vi "Measurement UI.vi"() -> ()   [LabVIEW 2023, in "FPT_SParam_VST UI.lvlib"]
uses:
  FPT_SParam_VST UI.lvlib
panel:
  in  "Tab Control 2":T1(tab)
  out "General Graph 1":T2(graph)
  out "General Graph 2":T2(graph)
  in  "Power sequencing file validity check":bool
  in  "Type of Stimulus":enum32{"CW", "Pulsed CW"}(ring)
  in  "Through Adapter S2P":string
  in  "Load S1P":string
  in  "Open S1P":string
  in  "Short S1P":string
  in  "Save Calibration File at":string
  in  "Calibration File Path":string
  in  "RFSG attenuation mode":enum32{"<None>", "Constant Attenuation"}(ring)=enum."Constant Attenuation"
  in  "RF In Switch":string
  in  "RF Out Switch":string
  in  "SnP File Path":string caption="SnP File Path (String)"
  in  "VST Resource Name":string="5842_0"
  in  "Power sequencing file path":string
  out "All Graph Refs":refnum<vi>[](array[refnum])
  out "S-Param Magnitude":dbl[][](array[numeric])
  out "S-Param Phase":dbl[][](array[numeric])
  out "S-Param":dbl[][](array[numeric])
  out "MeasTable":string[][](table)
  in  "Configuration":T3(ring)
  in  "Tab Control":T4(tab)
  in  "Power sequencing file path_update":path caption="Power Sequencing File Path"
  in  "Port2 Test":string
  in  "Port2 Reference":string
  in  "Port1 Test":string
  in  "Port1 Reference":string
  in  "RF In Switch_update":refnum<k15> caption="RF In Switch"
  in  "Port2 Incident":string
  in  "Port1 Incident":string
  in  "Common RFout":string
  in  "RF Out Switch_update":refnum<k15> caption="RF Out Switch"
  in  "Tab Control 3":enum32{"Calibrate", "Measure"}(tab)
  in  "Save Calibration Result_path":path caption="Save Calibration Result"
  in  "Short S1P_path":path caption="Short S1P"
  in  "Open S1P_path":path caption="Open S1P"
  in  "Load S1P_path":path caption="Load S1P"
  in  "Through Adapter S2P_path":path caption="Through Adapter S2P"
  in  "Calibration File Path_path":path caption="Calibration File Path"
  in  "RFSG attenuation mode_tab":enum32{"<None>", "Constant Attenuation"}(tab)=enum."Constant Attenuation" caption="RFSG Attenuation Mode"
  in  "RFSG external attenuation (dB)":dbl caption="External Attenuation" format="%#.3pdB"
  in  "VST name_update":refnum<k15> caption="VST Name"
  in  "RFSG port":string(combo)="port1" caption="RFSG Port"
  in  "RFmx port":string(combo)="port2" caption="RFmx Port"
  in  "SnP File Path_path":path caption="SnP File Path"
  in  "Step Size (Hz)":dbl=200.0 caption="Step Size" format="%#pHz"
  in  "Start Frequency (Hz)":dbl=4000000000.0 caption="Start Frequency" format="%#pHz"
  in  "Stop Frequency (Hz)":dbl=26000000000.0 caption="Stop Frequency" format="%#pHz"
  in  "IF Bandwidth (Hz)":dbl=100000.0 caption="IF Bandwidth" format="%#pHz"
  in  "External Gain (dB)":dbl caption="External Gain" format="%#fdB"
  in  "Power Level (dBm)":dbl=-10.0 caption="Power Level" format="%#fdBm"
  in  "Stimulus_tab":enum32{"CW", "Pulsed CW"}(tab)=enum."Pulsed CW" caption="Stimulus"
  in  "PRI (s)":dbl caption="PRI" format="%#.3ps"
  in  "Pulse Width (s)":dbl caption="Pulse Width" format="%#.3ps"
  in  "Average Mode":enum32{"Per Sweep", "Per Point"}(ring)
  in  "Number of Averages":i32=200
  in  "Action":enum32{"Calibrate", "Measure"}(ring)=enum."Measure"
  out "Status":string
  # "RFOut Switches"
  # "RFIn Switches"
  # "Calibration"
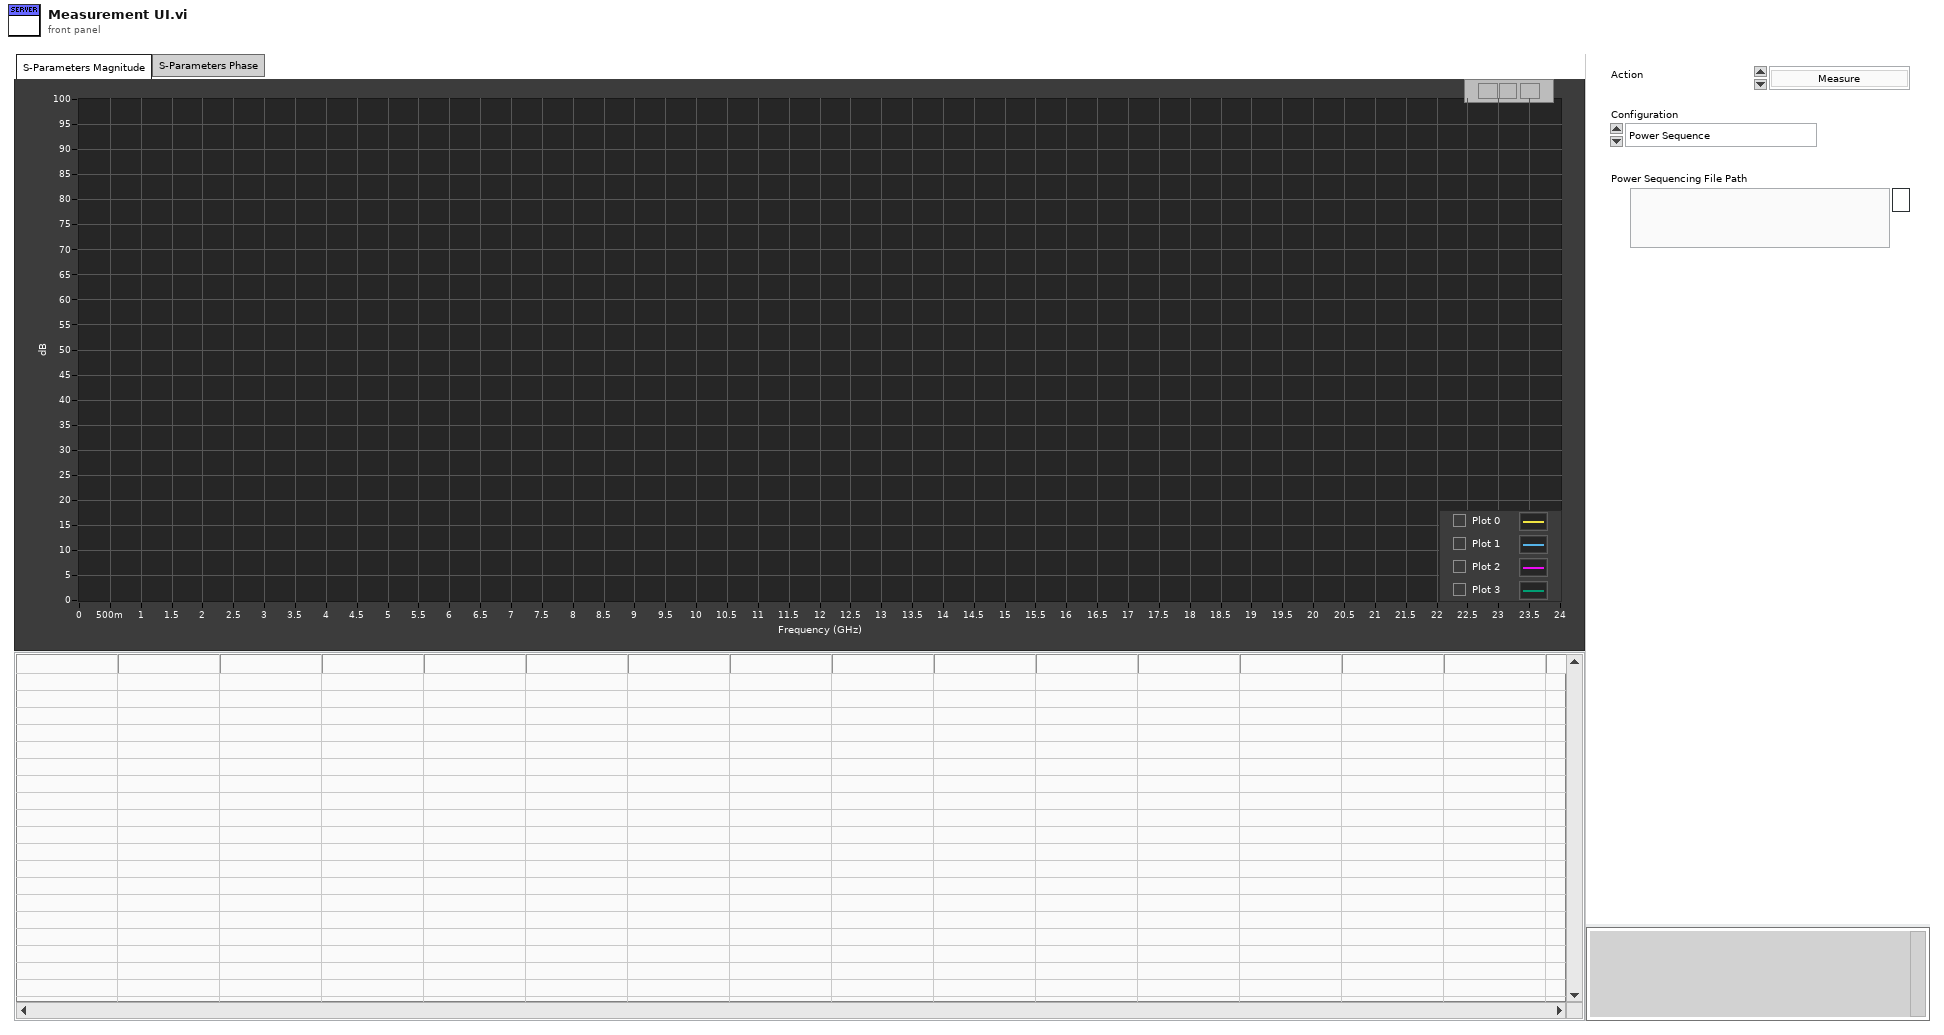
[diagram p1: front panel]
types:
  T1 = enum32{"S-Parameters Magnitude", "S-Parameters Phase", "Hiden Controls"}
  T2 = cluster{"Load currents":dbl[], "Efficiency":dbl[]}[]
  T3 = enum32{"Power Sequence", "Switches", "HW + Correction", "Measurement 1"}
  T4 = enum32{"Power Sequence", "Switches", "Correction", "Measurement 1"}
  T5 = cluster{"Shift":bool, "Ctrl":bool, "Alt":bool, "Cmd":bool, "Opt":bool}
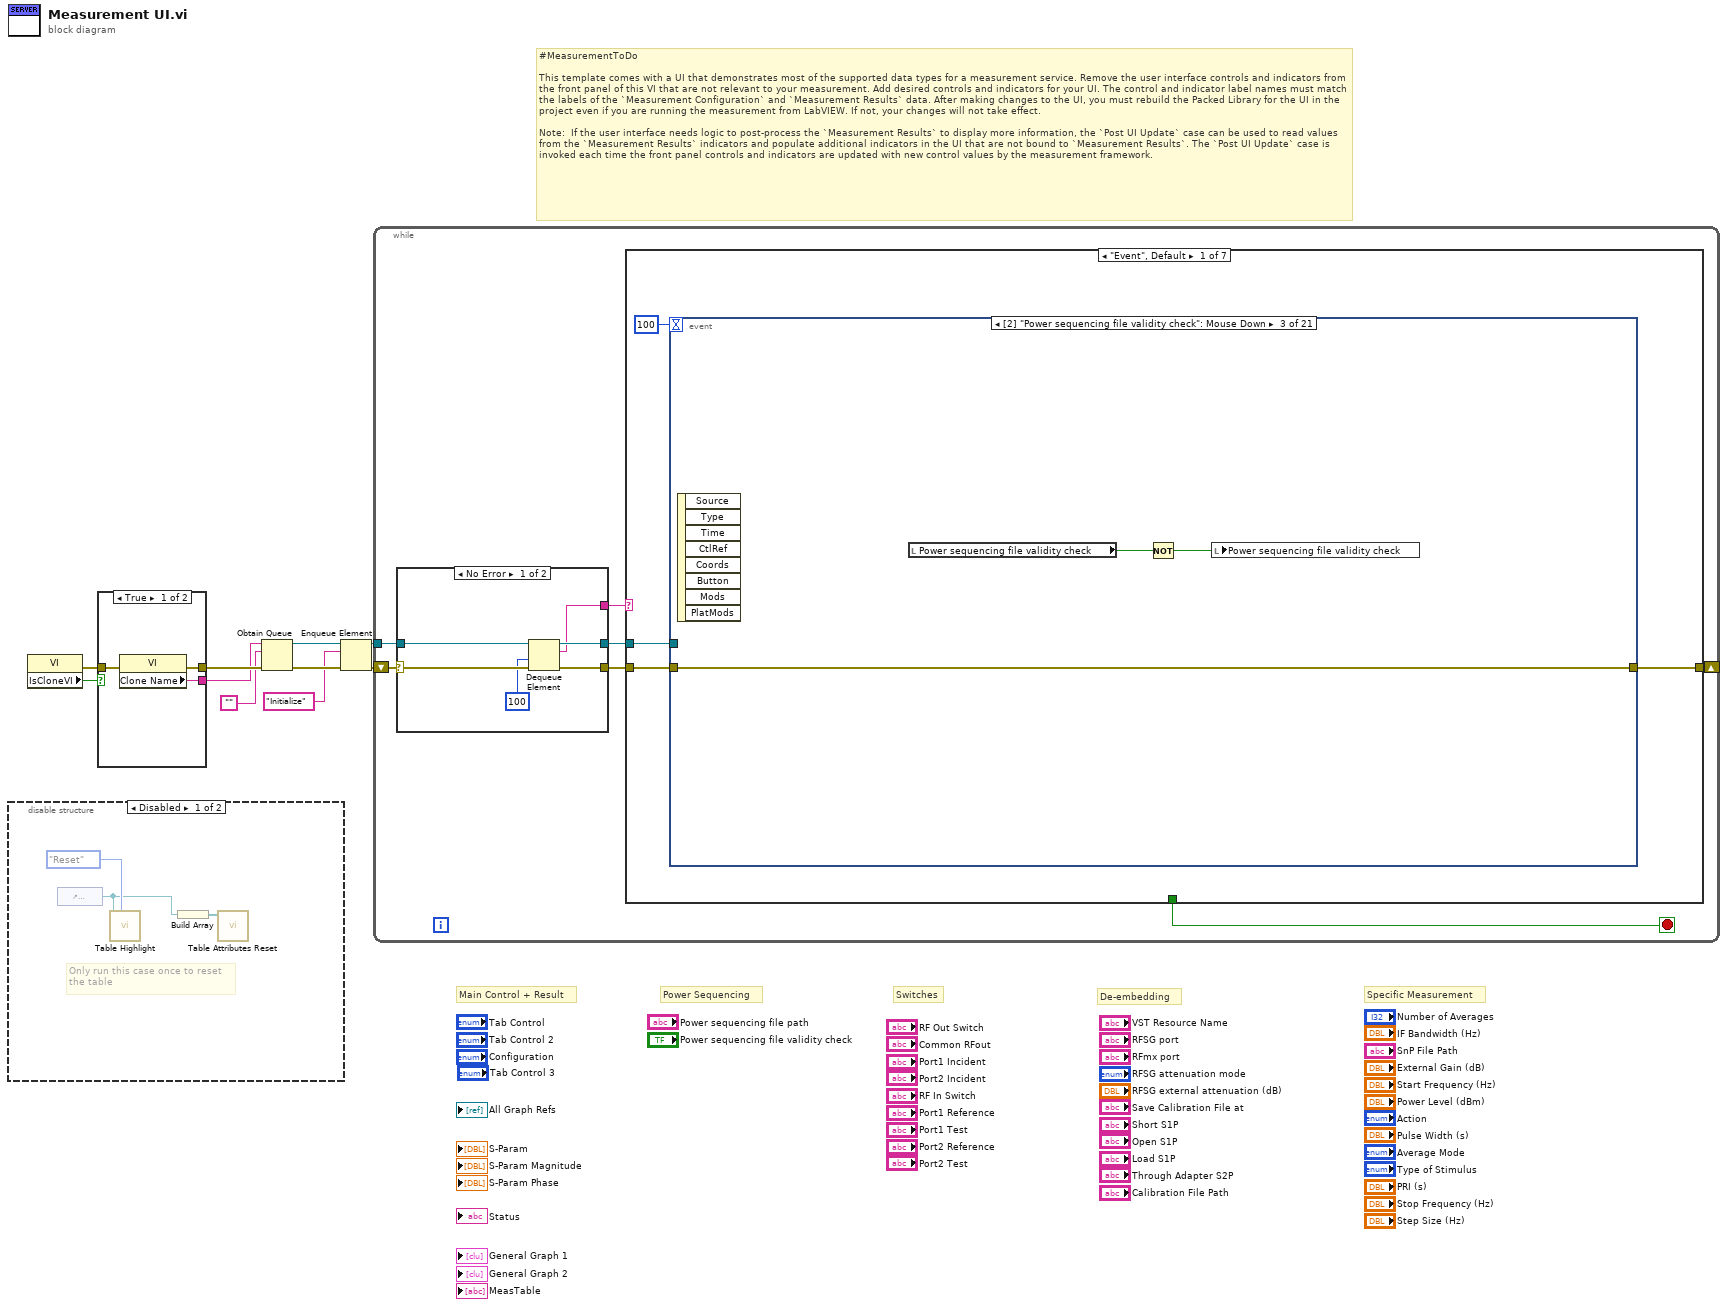
[diagram p0: block diagram]
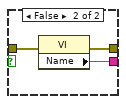
[diagram p3: hidden frame]
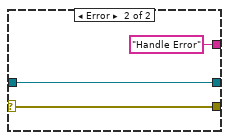
[diagram p4: hidden frame]
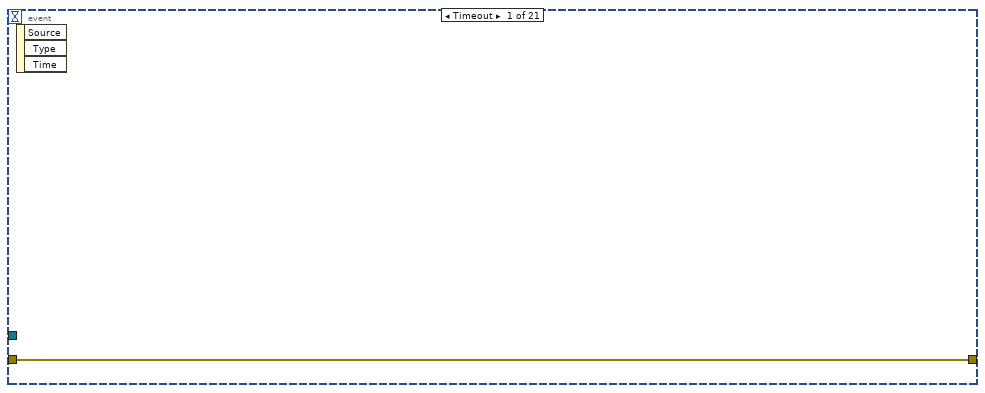
[diagram p5: hidden frame]
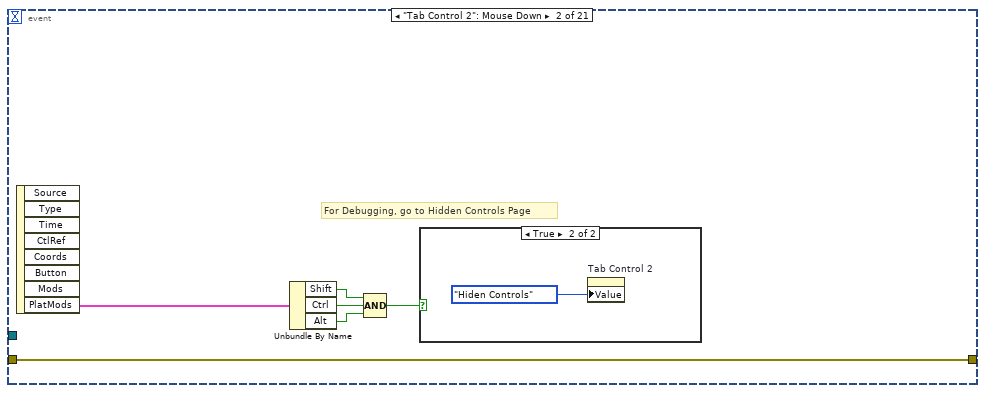
[diagram p6: hidden frame]
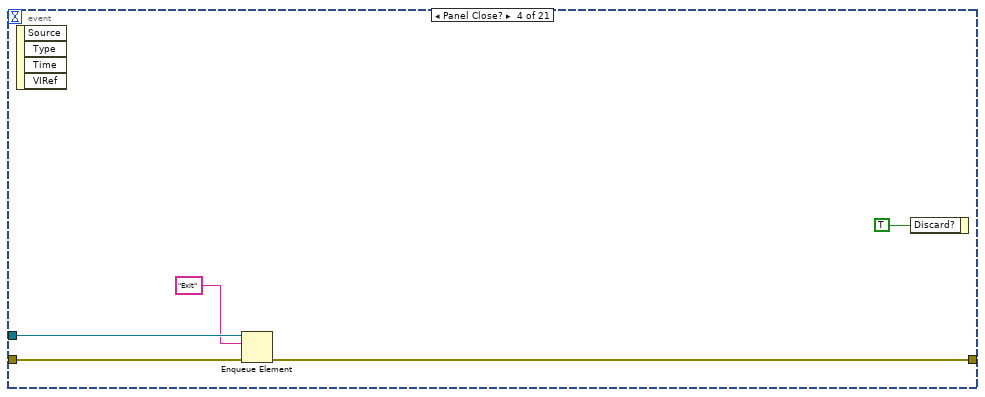
[diagram p8: hidden frame]
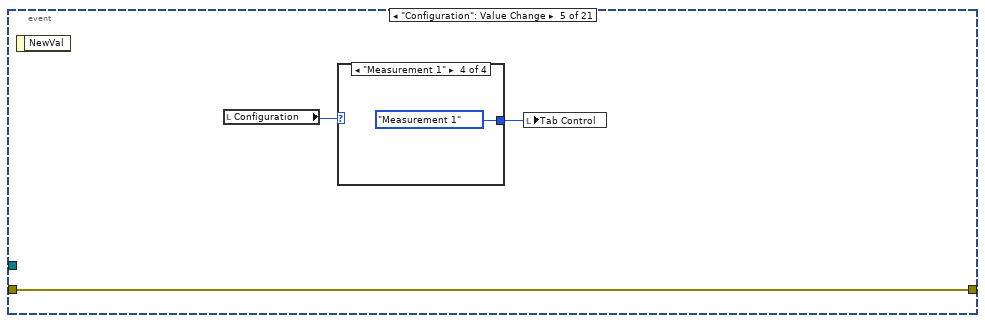
[diagram p9: hidden frame]
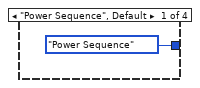
[diagram p10: hidden frame]
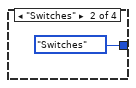
[diagram p11: hidden frame]
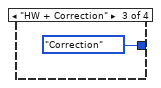
[diagram p12: hidden frame]
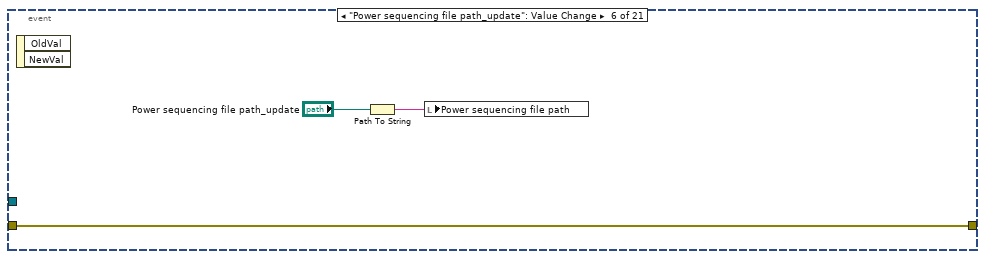
[diagram p13: hidden frame]
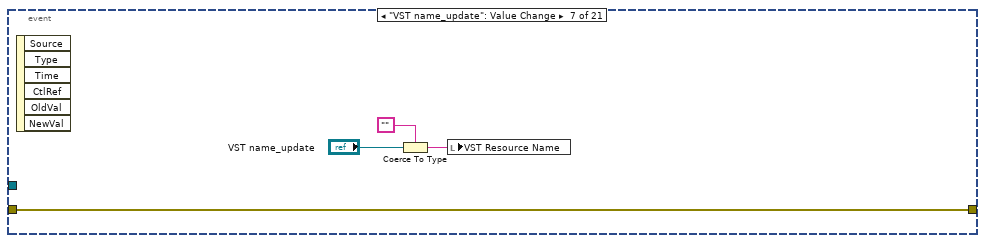
[diagram p14: hidden frame]
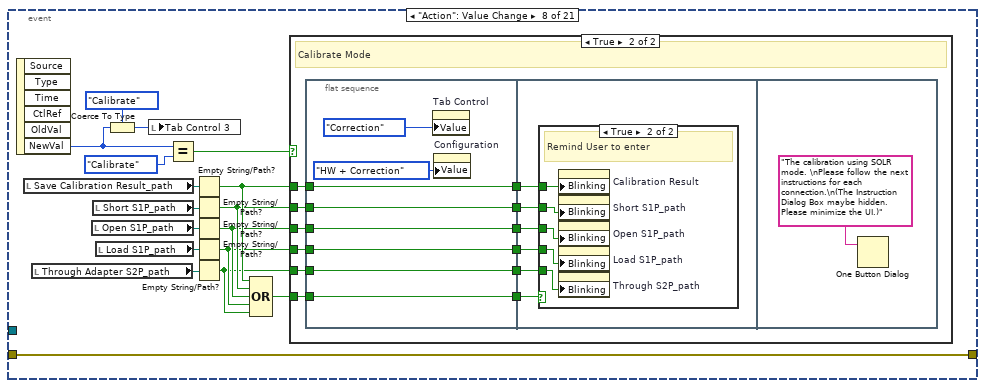
[diagram p15: hidden frame]
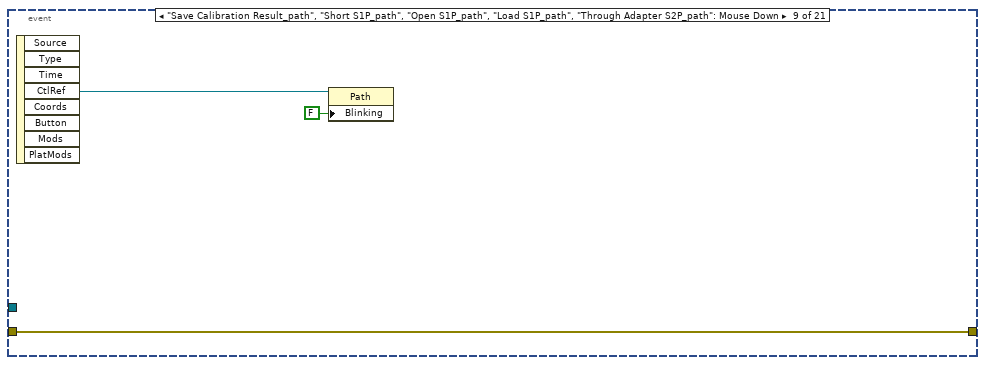
[diagram p18: hidden frame]
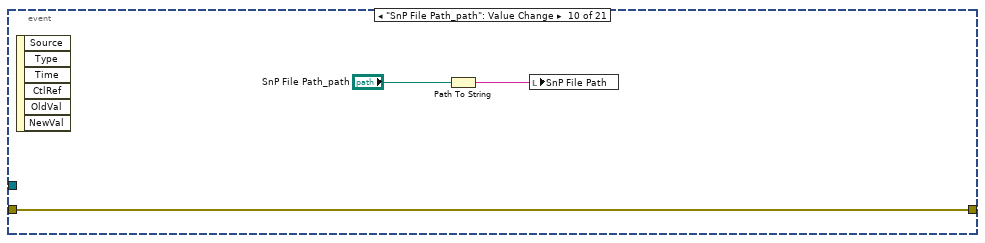
[diagram p19: hidden frame]
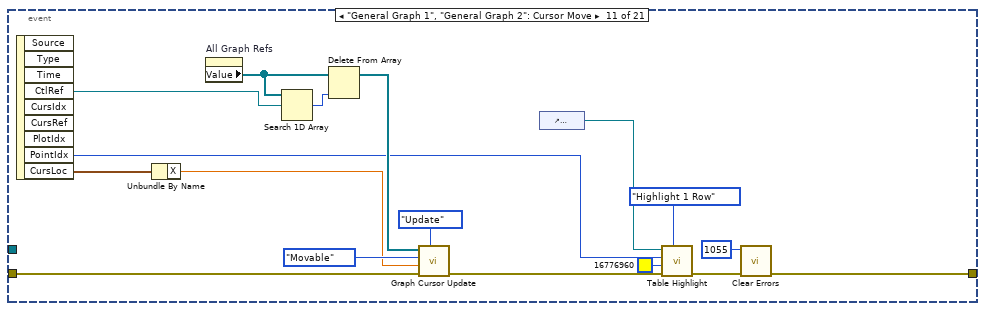
[diagram p20: hidden frame]
diagram:
  # "Switches"
  # "Specific Measurement"
  # "De-embedding"
  # "Power Sequencing"
  # "Main Control + Result"
  # "#MeasurementToDo  \n\nThis template comes with a UI that demonstrates most of the supported data types for a measurement service. Remove the user interface controls and indicators from the front panel of this VI that are not relevant to your measurement. Add desired controls and indicators for your UI. The control and indicator label names must match the labels of the `Measurement Configuration` and `Measurement Results` data. After making changes to the UI, you must rebuild the Packed Library for the UI in the project even if you are running the measurement from LabVIEW. If not, your changes will not take effect.\n\nNote:  If the user interface needs logic to post-process the `Measurement Results` to display more information, the `Post UI Update` case can be used to read values from the `Measurement Results` indicators and populate additional indicators in the UI that are not bound to `Measurement Results`. The `Post UI Update` case is invoked each time the front panel controls and indicators are updated with new control values by the measurement framework."
  n1 = disable-structure shown="Disabled" {
    frame Disabled {
      # "Only run this case once to reset\nthe table"
      n2 = control-ref of="MeasTable"() -> (w11:refnum<vi>)
      n3 = call "Table Highlight.vi"("Action"=enum16{"Reset", "Highlight 1 Row"}."Reset", "Table Ref in"=w11) -> ()  [unwired: 8 in, 2 out]
      n4 = Build Array(w11) -> (w12:refnum<vi>[])
      n5 = call "Table Attributes Reset.vi"("Table Refs"=w12) -> ()  [unwired: 11 in]
    }
    frame Enabled {
    }
  }
  n6 = property class="VI"() -> (error out=w1:errorcluster, "IsCloneVI"=w2:bool)  [unwired: 2 in, 1 out]
  n7 = case shown="True" w2 {
    tunnel: [w16 w19] -> w10
    tunnel: [w15 w18] -> w9
    tunnel: w1 -> [w14 w17]
    frame True {
      n8 = property class="VI"(error in=w14) -> (error out=w16:errorcluster, "Clone Name"=w15:string)  [unwired: 1 in, 1 out]
    }
    frame False {
      n9 = property class="VI"(error in=w17) -> (error out=w19:errorcluster, "Name"=w18:string)  [unwired: 1 in, 1 out]
    }
  }
  n10 = Obtain Queue(name (unnamed)=w9, element data type="", error in (no error)=w10) -> (queue out=w6:refnum<queue>, error out=w8:errorcluster)  [unwired: 2 in, 1 out]
  n11 = Enqueue Element(queue=w6, element="Initialize", error in (no error)=w8) -> (queue out=w5:refnum<queue>, error out=w7:errorcluster)  [unwired: 1 in, 1 out]
  n12 = while {
    shift-right: [w21] -> _
    shift-left: w7 -> [w26]
    tunnel: w5 -> [w24]
    stop <- w20 stop-if-true
    n13 = case shown="No Error" w26 {
      selector: w26 -> [w32 w35]
      tunnel: [w31 w35] -> w25
      tunnel: w24 -> [w30 w34]
      tunnel: [w29 w34] -> w23
      tunnel: [w28 "Handle Error"] -> w22
      frame No Error {
        n14 = Dequeue Element(queue=w30, timeout in ms (-1)=100, error in (no error)=w32) -> (queue out=w29:refnum<queue>, element=w28:string, error out=w31:errorcluster)  [unwired: 1 out]
      }
      frame Error {
      }
    }
    n15 = case shown="\"Event\", Default" w22 {
      tunnel: w25 -> [w38 w182 w219 w236 w247 w254 w255]
      tunnel: w23 -> [w36 _ w218 w235 _ w252 _]
      tunnel: [w39 w182 w219 w237 w246 w249 w255] -> w21
      tunnel: [_ _ _ _ _ TRUE _] -> w20
      frame "Event", Default {
        n16 = event shown="[2] \"Power sequencing file validity check\": Mouse Down" {
          selector: _ -> [_ _ _ _ _ _ _ _ _ _ _ _ _ _ _ _ _ _ _ _ _]
          dyn-events: _ -> [_ _ _ _ _ _ _ _ _ _ _ _ _ _ _ _ _ _ _ _ _]
          timeout: 100 -> [_ _ _ _ _ _ _ _ _ _ _ _ _ _ _ _ _ _ _ _ _]
          tunnel: [w40 w46 w50 w53 w58 w63 w66 w86 w121 w124 w134 w145 w149 w153 w156 w159 w162 w165 w168 w171 w175] -> w39
          tunnel: w38 -> [w40 w46 w50 w54 w58 w63 w66 w86 w121 w124 w135 w145 w149 w153 w156 w159 w162 w165 w168 w171 w175]
          tunnel: w36 -> [_ _ _ w52 _ _ _ _ _ _ _ _ _ _ _ _ _ _ _ _ _]
          event Timeout {
            n17 = event-data() -> ()  [unwired: 1 in, 3 out]
          }
          event "Tab Control 2": Mouse Down {
            # "For Debugging, go to Hidden Controls Page"
            n18 = event-data() -> ("PlatMods"=w45:T5)  [unwired: 1 in, 7 out]
            n19 = Unbundle By Name(w45) -> ("Shift"=w44:bool, "Ctrl"=w43:bool, "Alt"=w42:bool)
            n20 = Compound Arithmetic op=AND(w44, w43, w42) -> (w41:bool)
            n21 = case shown="True" w41 {
              frame False {
              }
              frame True {
                n22 = property on="Tab Control 2" class="TabCtl (strict)"("Value"=T1."Hiden Controls" ("Tab Control 2")) -> ()  [unwired: 2 in, 2 out]
              }
            }
          }
          event "Power sequencing file validity check": Mouse Down {
            n23 = event-data() -> ()  [unwired: 1 in, 8 out]
            n24 = local read "Power sequencing file validity check"() -> (w49:bool)
            n25 = Not(x=w49) -> (.not. x?=w48:bool)
            n26 = local write "Power sequencing file validity check"(w48) -> ()
          }
          event Panel Close? {
            n27 = event-data() -> ()  [unwired: 1 in, 4 out]
            n28 = Enqueue Element(queue=w52, element="Exit", error in (no error)=w54) -> (error out=w53:errorcluster)  [unwired: 1 in, 2 out]
            n29 = event-data("Discard?"=TRUE) -> ()  [unwired: 1 in, 1 out]
          }
          event "Configuration": Value Change {
            n30 = event-data() -> ()  [unwired: 1 in, 1 out]
            n31 = local read "Configuration"() -> (w56:T3)
            n32 = case shown="\"Measurement 1\"" w56 {
              tunnel: [T4."Power Sequence" ("Tab Control") T4."Switches" ("Tab Control") T4."Correction" ("Tab Control") T4."Measurement 1" ("Tab Control")] -> w57
              frame "Power Sequence", Default {
              }
              frame "Switches" {
              }
              frame "HW + Correction" {
              }
              frame "Measurement 1" {
              }
            }
            n33 = local write "Tab Control"(w57) -> ()
          }
          event "Power sequencing file path_update": Value Change {
            n34 = event-data() -> ()  [unwired: 1 in, 2 out]
            n35 = Path To String(path="Power sequencing file path_update") -> (string=w64:string)
            n36 = local write "Power sequencing file path"(w64) -> ()
          }
          event "VST name_update": Value Change {
            n37 = event-data() -> ()  [unwired: 1 in, 6 out]
            n38 = Coerce To Type(0:"VST name_update", 1:"") -> (2:w68:string)
            n39 = local write "VST Resource Name"(w68) -> ()
          }
          event "Action": Value Change {
            n40 = event-data() -> ("NewVal"=w83:enum32{"Calibrate", "Measure"})  [unwired: 1 in, 5 out]
            n41 = local read "Save Calibration Result_path"() -> (w80:path)
            n42 = local read "Through Adapter S2P_path"() -> (w76:path)
            n43 = local read "Open S1P_path"() -> (w78:path)
            n44 = local read "Short S1P_path"() -> (w79:path)
            n45 = local read "Load S1P_path"() -> (w77:path)
            n46 = Coerce To Type(0:w83, 1:enum32{"Calibrate", "Measure"}."Calibrate" ("Tab Control 3")) -> (2:w81:enum32{"Calibrate", "Measure"})
            n47 = local write "Tab Control 3"(w81) -> ()
            n48 = Equal?(x=w83, y=enum32{"Calibrate", "Measure"}."Calibrate") -> (x = y?=w84:bool)
            n49 = Empty String/Path?(string/path=w80) -> (empty?=w75:bool)
            n50 = Empty String/Path?(string/path=w79) -> (empty?=w74:bool)
            n51 = Empty String/Path?(string/path=w78) -> (empty?=w73:bool)
            n52 = Empty String/Path?(string/path=w77) -> (empty?=w72:bool)
            n53 = Empty String/Path?(string/path=w76) -> (empty?=w71:bool)
            n54 = Compound Arithmetic op=OR(w75, w74, w73, w72, w71) -> (w70:bool)
            n55 = case shown="True" w84 {
              tunnel: w75 -> [_ w97]
              tunnel: w74 -> [_ w95]
              tunnel: w73 -> [_ w93]
              tunnel: w72 -> [_ w91]
              tunnel: w71 -> [_ w89]
              tunnel: w70 -> [_ w87]
              frame False {
                # "Measure Mode"
              }
              frame True {
                # "Calibrate Mode"
                n56 = flat-sequence {
                  tunnel: [w105] -> w98
                  tunnel: w97 -> [w105]
                  tunnel: [w104] -> w96
                  tunnel: w95 -> [w104]
                  tunnel: [w103] -> w94
                  tunnel: w93 -> [w103]
                  tunnel: [w102] -> w92
                  tunnel: w91 -> [w102]
                  tunnel: [w101] -> w90
                  tunnel: w89 -> [w101]
                  tunnel: [w100] -> w88
                  tunnel: w87 -> [w100]
                  tunnel: w98 -> [w112]
                  tunnel: w96 -> [w111]
                  tunnel: w94 -> [w110]
                  tunnel: w92 -> [w109]
                  tunnel: w90 -> [w108]
                  tunnel: w88 -> [w107]
                  frame #0 {
                    n57 = property on="Tab Control" class="TabCtl (strict)"("Value"=T4."Correction" ("Tab Control")) -> ()  [unwired: 2 in, 2 out]
                    n58 = property on="Configuration" class="Enum (strict)"("Value"=T3."HW + Correction" ("Configuration")) -> ()  [unwired: 2 in, 2 out]
                  }
                  frame #1 {
                    n59 = case shown="True" w107 {
                      tunnel: w112 -> [_ w117]
                      tunnel: w111 -> [_ w116]
                      tunnel: w110 -> [_ w115]
                      tunnel: w109 -> [_ w114]
                      tunnel: w108 -> [_ w113]
                      frame False {
                      }
                      frame True {
                        # "Remind User to enter"
                        n60 = property on="Calibration Result" class="Path"("Blinking"=w117) -> ()  [unwired: 2 in, 2 out]
                        n61 = property on="Short S1P_path" class="Path"("Blinking"=w116) -> ()  [unwired: 2 in, 2 out]
                        n62 = property on="Open S1P_path" class="Path"("Blinking"=w115) -> ()  [unwired: 2 in, 2 out]
                        n63 = property on="Load S1P_path" class="Path"("Blinking"=w114) -> ()  [unwired: 2 in, 2 out]
                        n64 = property on="Through S2P_path" class="Path"("Blinking"=w113) -> ()  [unwired: 2 in, 2 out]
                      }
                    }
                  }
                  frame #2 {
                    n65 = One Button Dialog(message="The calibration using SOLR mode. \nPlease follow the next instructions for each connection.\n(The Instruction Dialog Box maybe hidden. Please minimize the UI.)") -> ()  [unwired: 1 in, 1 out]
                  }
                }
              }
            }
          }
          event "Save Calibration Result_path", "Short S1P_path", "Open S1P_path", "Load S1P_path", "Through Adapter S2P_path": Mouse Down {
            n66 = event-data() -> ("CtlRef"=w120:refnum<vi>)  [unwired: 1 in, 7 out]
            n67 = property class="Path"(reference=w120, "Blinking"=FALSE) -> ()  [unwired: 1 in, 2 out]
          }
          event "SnP File Path_path": Value Change {
            n68 = event-data() -> ()  [unwired: 1 in, 6 out]
            n69 = Path To String(path="SnP File Path_path") -> (string=w122:string)
            n70 = local write "SnP File Path"(w122) -> ()
          }
          event "General Graph 1", "General Graph 2": Cursor Move {
            n71 = event-data() -> ("CtlRef"=w125:refnum<vi>, "PointIdx"=w128:i32, "CursLoc"=w133:cluster{"X":dbl, "Y":dbl})  [unwired: 1 in, 6 out]
            n72 = Unbundle By Name(w133) -> ("X"=w132:dbl)
            n73 = property on="All Graph Refs" class="Arr (strict)"() -> ("Value"=w129:refnum<vi>[])  [unwired: 2 in, 2 out]
            n74 = Search 1D Array(1D array=w129, element=w125) -> (index of element=w131:i32)  [unwired: 1 in]
            n75 = Delete From Array(array=w129, index=w131) -> (array with subset deleted=w130:refnum<vi>[])  [unwired: 1 in, 1 out]
            n76 = call "Graph Cursor Update.vi"("Action"=enum16{"Reset", "Update"}."Update" ("Cursor to Update"), "error in"=w135, "New X position"=w132, "Cursor Type"=enum16{"Movable", "Fixed", "All"}."Movable", "Graph Refs in"=w130) -> ("error out"=w138:errorcluster)  [unwired: 5 in, 1 out]
            n77 = control-ref of="MeasTable"() -> (w127:refnum<vi>)
            n78 = call "Table Highlight.vi"("Action"=enum16{"Reset", "Highlight 1 Row"}."Highlight 1 Row", "error in"=w138, "Color Box"=u32 16776960, "Row"=w128, "Table Ref in"=w127) -> ("error out"=w140:errorcluster)  [unwired: 5 in, 1 out]
            n79 = call <vilib>:"Clear Errors.vi"("error in (no error)"=w140, "specific error code to clear (0: all)"=1055) -> ("error out"=w134:errorcluster)  [unwired: 4 in, 1 out]
          }
          event "RF Out Switch_update": Value Change {
            n80 = event-data() -> ()  [unwired: 1 in, 6 out]
            n81 = Coerce To Type(0:"RF Out Switch_update", 1:"") -> (2:w143:string)
            n82 = local write "RF Out Switch"(w143) -> ()
          }
          event "RF In Switch_update": Value Change {
            n83 = event-data() -> ()  [unwired: 1 in, 6 out]
            n84 = Coerce To Type(0:"RF In Switch_update", 1:"") -> (2:w147:string)
            n85 = local write "RF In Switch"(w147) -> ()
          }
          event "RFSG attenuation mode_tab": Value Change {
            n86 = event-data() -> ()  [unwired: 1 in, 6 out]
            n87 = Coerce To Type(0:"RFSG attenuation mode_tab", 1:enum32{"<None>", "Constant Attenuation"}."<None>" ("RFSG attenuation mode")) -> (2:w151:enum32{"<None>", "Constant Attenuation"})
            n88 = local write "RFSG attenuation mode"(w151) -> ()
          }
          event "Save Calibration Result_path": Value Change {
            n89 = event-data() -> ()  [unwired: 1 in, 6 out]
            n90 = Path To String(path="Save Calibration Result_path") -> (string=w154:string)
            n91 = local write "Save Calibration File at"(w154) -> ()
          }
          event "Short S1P_path": Value Change {
            n92 = event-data() -> ()  [unwired: 1 in, 6 out]
            n93 = Path To String(path="Short S1P_path") -> (string=w158:string)
            n94 = local write "Short S1P"(w158) -> ()
          }
          event "Open S1P_path": Value Change {
            n95 = event-data() -> ()  [unwired: 1 in, 6 out]
            n96 = Path To String(path="Open S1P_path") -> (string=w161:string)
            n97 = local write "Open S1P"(w161) -> ()
          }
          event "Load S1P_path": Value Change {
            n98 = event-data() -> ()  [unwired: 1 in, 6 out]
            n99 = Path To String(path="Load S1P_path") -> (string=w164:string)
            n100 = local write "Load S1P"(w164) -> ()
          }
          event "Through Adapter S2P_path": Value Change {
            n101 = event-data() -> ()  [unwired: 1 in, 6 out]
            n102 = Path To String(path="Through Adapter S2P_path") -> (string=w167:string)
            n103 = local write "Through Adapter S2P"(w167) -> ()
          }
          event "Calibration File Path_path": Value Change {
            n104 = event-data() -> ()  [unwired: 1 in, 6 out]
            n105 = Path To String(path="Calibration File Path_path") -> (string=w170:string)
            n106 = local write "Calibration File Path"(w170) -> ()
          }
          event "Stimulus_tab": Value Change {
            n107 = event-data() -> ()  [unwired: 1 in, 6 out]
            n108 = Coerce To Type(0:"Stimulus_tab", 1:enum16{"CW", "Pulsed CW"}."CW" ("Type of Stimulus")) -> (2:w172:enum16{"CW", "Pulsed CW"})
            n109 = local write "Type of Stimulus"(w172) -> ()
          }
        }
      }
      frame "Initialize" {
        w176 = enum32{"Calibrate", "Measure"}."Measure" ("Action")
        w177 = 0
        n110 = control-ref of="General Graph 1"() -> (w180:refnum<vi>)
        n111 = control-ref of="General Graph 2"() -> (w178:refnum<vi>)
        n112 = local write "Tab Control"(w177) -> ()
        n113 = local write "Configuration"(w177) -> ()
        n114 = local write "Tab Control 2"(w177) -> ()
        n115 = local write "Action"(w176) -> ()
        n116 = local write "Tab Control 3"(w176) -> ()
        n117 = Build Array(w180, w178) -> (w179:refnum<vi>[])
        n118 = property on="All Graph Refs" class="Arr (strict)"("Value"=w179) -> ()  [unwired: 2 in, 2 out]
        n119 = call "Graph Set Cursor Mode.vi"("Cursor Mode"=enum32{"Free-Drag", "Single-Plot", "Multi-Plot"}."Multi-Plot", "Graph Refs in"=w179) -> ()  [unwired: 8 in, 2 out]
      }
      frame "Post UI Update" {
        # "This case will be triggered, after framework updates the User interface with result values.\nUsed to update data type def"
        n120 = local read "Power sequencing file path"() -> (w215:string)
        n121 = local read "Save Calibration File at"() -> (w209:string)
        n122 = local read "Through Adapter S2P"() -> (w189:string)
        n123 = local read "Calibration File Path"() -> (w186:string)
        n124 = local read "SnP File Path"() -> (w208:string)
        n125 = Enqueue Element(queue=w218, element="Post UI Update 2") -> ()  [unwired: 2 in, 3 out]
        n126 = local read "Open S1P"() -> (w205:string)
        n127 = local read "Short S1P"() -> (w214:string)
        n128 = local read "Load S1P"() -> (w190:string)
        n129 = String To Path(string=w190) -> (path=w191:path)
        n130 = String To Path(string=w189) -> (path=w188:path)
        n131 = String To Path(string=w186) -> (path=w187:path)
        n132 = String To Path(string=w215) -> (path=w216:path)
        n133 = String To Path(string=w209) -> (path=w206:path)
        n134 = String To Path(string=w208) -> (path=w207:path)
        n135 = String To Path(string=w205) -> (path=w204:path)
        n136 = String To Path(string=w214) -> (path=w213:path)
        n137 = local write "Power sequencing file path_update"(w216) -> ()
        n138 = local write "Save Calibration Result_path"(w206) -> ()
        n139 = local write "SnP File Path_path"(w207) -> ()
        n140 = local write "Open S1P_path"(w204) -> ()
        n141 = local write "Short S1P_path"(w213) -> ()
        n142 = local write "Load S1P_path"(w191) -> ()
        n143 = local write "Through Adapter S2P_path"(w188) -> ()
        n144 = local write "Calibration File Path_path"(w187) -> ()
        n145 = local read "RFSG attenuation mode"() -> (w197:enum32{"<None>", "Constant Attenuation"})
        n146 = local read "VST Resource Name"() -> (w210:string)
        n147 = local read "Type of Stimulus"() -> (w193:enum32{"CW", "Pulsed CW"})
        n148 = local read "RF Out Switch"() -> (w203:string)
        n149 = local read "RF In Switch"() -> (w198:string)
        n150 = local read "Action"() -> (w184:enum32{"Calibrate", "Measure"})
        n151 = Coerce To Type(0:w203, 1:refnum<k15> refnum ("RFSG name_update")) -> (2:w201:refnum<k15>)
        n152 = Coerce To Type(0:w198, 1:refnum<k15> refnum ("RFSG name_update")) -> (2:w200:refnum<k15>)
        n153 = Coerce To Type(0:w184, 1:enum32{"Calibrate", "Measure"}."Calibrate" ("Tab Control 3")) -> (2:w183:enum32{"Calibrate", "Measure"})
        n154 = Coerce To Type(0:w210, 1:refnum<k15> refnum ("RFSG name_update")) -> (2:w212:refnum<k15>)
        n155 = Coerce To Type(0:w197, 1:enum32{"<None>", "Constant Attenuation"}."Constant Attenuation" ("RFSG attenuation mode_tab")) -> (2:w196:enum32{"<None>", "Constant Attenuation"})
        n156 = Coerce To Type(0:w193, 1:enum32{"CW", "Pulsed CW"}."CW" ("Stimulus_tab")) -> (2:w194:enum32{"CW", "Pulsed CW"})
        n157 = local write "RF Out Switch_update"(w201) -> ()
        n158 = local write "RFSG attenuation mode_tab"(w196) -> ()
        n159 = local write "VST name_update"(w212) -> ()
        n160 = local write "RF In Switch_update"(w200) -> ()
        n161 = local write "Stimulus_tab"(w194) -> ()
        n162 = local write "Tab Control 3"(w183) -> ()
      }
      frame "Post UI Update 2" {
        w221 = string[] ["S11(deg)", "S21(deg)", "S12(deg)", "S22(deg)"] ("Plot Names")
        w222 = string[] ["S11(dB)", "S21(dB)", "S12(dB)", "S22(dB)"] ("Plot Names")
        # "Phase Graph"
        # "Mag Graph"
        # "Run after Post UI Update. Can be duplicate is need more processing.\nUtilize this case to convert the result to graph or table"
        n163 = Enqueue Element(queue=w235, element="Post UI Update 3", error in (no error)=w236) -> (error out=w237:errorcluster)  [unwired: 1 in, 2 out]
        n164 = control-ref of="General Graph 1"() -> (w234:refnum<vi>)
        n165 = property on="S-Param Magnitude" class="Arr (strict)"() -> ("Value"=w231:dbl[][])  [unwired: 2 in, 2 out]
        n166 = control-ref of="General Graph 2"() -> (w232:refnum<vi>)
        n167 = property on="S-Param Phase" class="Arr (strict)"() -> ("Value"=w228:dbl[][])  [unwired: 2 in, 2 out]
        n168 = call "Graph Assign Plot Names and Data.vi"("Legend Number of Rows"=4, "X Ys Data"=w231, "Plot Names"=w222, "Graph Ref in"=w234) -> ()  [unwired: 5 in, 3 out]
        n169 = call "Graph Assign Plot Names and Data.vi"("Legend Number of Rows"=4, "X Ys Data"=w228, "Plot Names"=w221, "Graph Ref in"=w232) -> ()  [unwired: 5 in, 3 out]
        n170 = Interleave 1D Arrays(w222, w221) -> (w220:string[])
        n171 = Build Array (concatenate)("Frequency (GHz)" ("S-Parameter"), w220) -> (w223:string[])
        n172 = for {
          tunnel: w231 -> [w241] mode=indexing
          tunnel: w228 -> [w240] mode=indexing
          tunnel: [w239] -> w229 mode=concatenating
          n173 = Build Array(w241, w240) -> (w239:dbl[][])
        }
        n174 = control-ref of="MeasTable"() -> (w233:refnum<vi>)
        n175 = Delete From Array(array=w229, index (row)=0 ("index")) -> (array with subset deleted=w227:dbl[][])  [unwired: 2 in, 1 out]
        n176 = call "Table Set Header Name and Data.vi"("Data"=w227, "Header"=w223, "Table Ref"=w233) -> ()  [unwired: 9 in]
      }
      frame "Post UI Update 3" {
        n177 = property on="All Graph Refs" class="Arr (strict)"() -> ("Value"=w243:refnum<vi>[])  [unwired: 2 in, 2 out]
        n178 = call "Graph Cursor Update.vi"("Action"=enum16{"Reset", "Update"}."Update", "error in"=w247, "New X position"=0.0, "Cursor Type"=enum16{"Movable", "Fixed", "All"}."Movable", "Graph Refs in"=w243) -> ("error out"=w246:errorcluster)  [unwired: 5 in, 1 out]
      }
      frame "Exit" {
        # "This case is triggered to close the User Interface from framework"
        n179 = Flush Queue(queue=w252, error in (no error)=w254) -> (queue out=w251:refnum<queue>, error out=w250:errorcluster)  [unwired: 1 out]
        n180 = Release Queue(queue=w251, force destroy? (F)=TRUE, error in (no error)=w250) -> (error out=w249:errorcluster)  [unwired: 2 out]
      }
      frame "Handle Error" {
      }
    }
  }
